vi "Fire Control.vi"(10 "ShooterDevRef":T14={"Frisbee Load Motor"={"DeviceStatus"={"status"=FALSE, "code"=0, "source"=""}, "Type"=enum."PWM", "PWM"={"Digital Module"=enum."Digital Module 1", "PWM Channel"=enum."Invalid", "DeadBand"={"Name"="", "maxPositivePwm"=0, "minPositivePwm"=0, "centerPwm"=0, "maxNegativePwm"=0, "minNegativePwm"=0, "angularRange"=0}}, "CAN"={"Device Number"=0, "Control Mode"=enum."Percent VBus", "Semaphore"=refnum, "Max Vout"=12.0}, "Invert"=FALSE, "TransformRef"=refnum, "InvTransformRef"=refnum}, "On Deck Sensor"={"DevStatus"={"status"=FALSE, "code"=0, "source"=""}, "DIO Channel"=enum."DIO 1", "Digital Module"=enum."Digital Module 1"}, "Load Sensor"={"DevStatus"={"status"=FALSE, "code"=0, "source"=""}, "DIO Channel"=enum."DIO 1", "Digital Module"=enum."Digital Module 1"}, "Front Sensor"={"DevStatus"={"status"=FALSE, "code"=0, "source"=""}, "DIO Channel"=enum."DIO 1", "Digital Module"=enum."Digital Module 1"}, "Firing Motors"={"DevStatus"={"status"=FALSE, "code"=0, "source"=""}, "Motors[]"=[], "Square Inputs"=FALSE, "Max Output"=1.0, "Isochronous"=FALSE}, "Piston"={"DevStatus"={"status"=FALSE, "code"=0, "source"=""}, "Relay Channel"=enum."Invalid", "Digital Module"=enum."Digital Module 1", "Relay Direction"=enum."Both directions"}}, 11 "Fire":bool) -> ()   [LabVIEW 2013]
uses:
  <vilib>/Rock Robotics/WPI/MotorControl/WPI_MotorControlDeviceRef.ctl
  <vilib>/Rock Robotics/SystemInterfaces/Typedef/FPGA_TypedefDigitalModule.ctl
  <vilib>/Rock Robotics/SystemInterfaces/DIO/FPGA_DIOPWMChannel.ctl
  <vilib>/Rock Robotics/WPI/PWM/WPI_PWMDeadband.ctl
  <vilib>/Rock Robotics/WPI/CAN/Jaguar/SubVIs/WPI_CANJaguar_ControlMode.ctl
  <vilib>/Rock Robotics/WPI/PWM/WPI_PWMTransform_ConPane.ctl
  <vilib>/Rock Robotics/WPI/DigitalInput/WPI_DigitalInputDevRef.ctl
  <vilib>/Rock Robotics/SystemInterfaces/DIO/FPGA_DIOChannel.ctl
  <vilib>/Rock Robotics/WPI/RobotDrive/WPI_RobotDriveDevRef.ctl
  <vilib>/Rock Robotics/WPI/Relay/WPI_RelayDevRef.ctl
  <vilib>/Rock Robotics/SystemInterfaces/DIO/FPGA_DIORelayChannel.ctl
  <vilib>/Rock Robotics/WPI/Relay/WPI_RelayDirection.ctl
  Utils/ShooterStateEnum.ctl
  <vilib>/Rock Robotics/WPI/Relay/WPI_RelayValue.ctl
panel:
  in  "Load Disk Time":dbl
  in  "Wheel Time":dbl
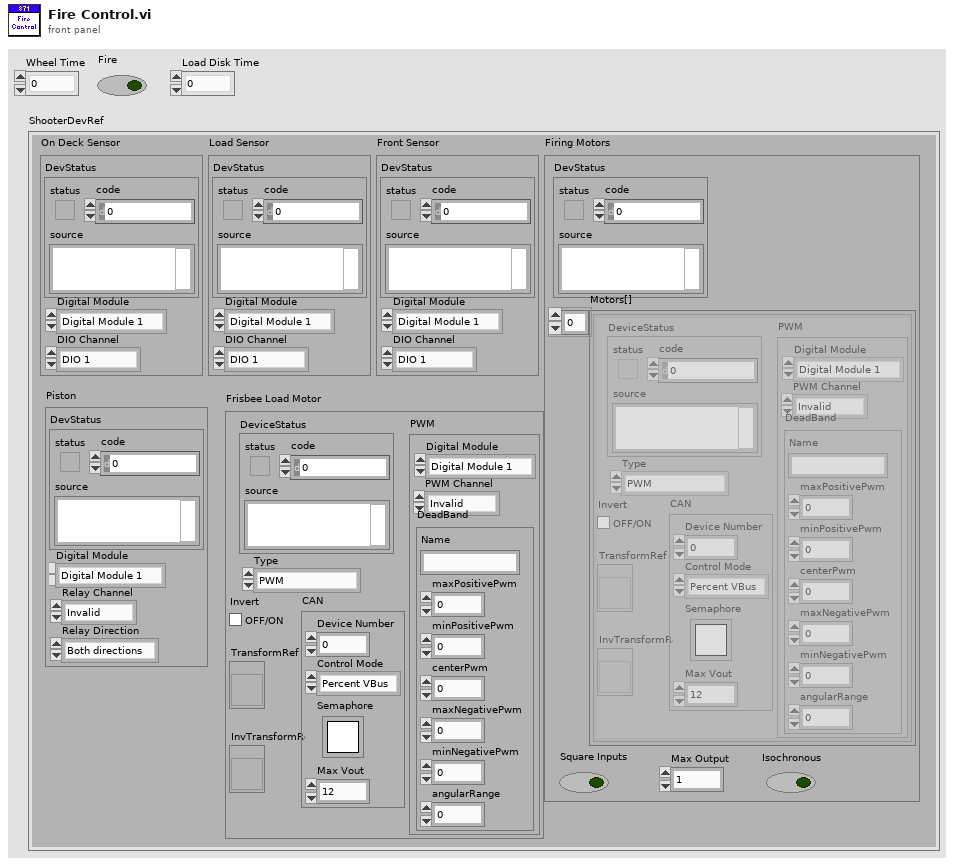
[diagram p1: front panel]
types:
  T1 = typedef "WPI_MotorControlDeviceRef.ctl" = cluster{"DeviceStatus":errorcluster, "Type":enum16{"PWM", "CAN"}, "PWM":cluster{"Digital Module":T2, "PWM Channel":T3, "DeadBand":T4}, "CAN":cluster{"Device Number":u8, "Control Mode":T5, "Semaphore":T6, "Max Vout":dbl}, "Invert":bool, "TransformRef":T7, "InvTransformRef":T7}
  T2 = typedef "FPGA_TypedefDigitalModule.ctl" = enum16{"Digital Module 1", "Digital Module 2"}
  T3 = typedef "FPGA_DIOPWMChannel.ctl" = enum8{"PWM 1", "PWM 2", "PWM 3", "PWM 4", "PWM 5", "PWM 6", "PWM 7", "PWM 8", "PWM 9", "PWM 10", "Invalid"}
  T4 = typedef "WPI_PWMDeadband.ctl" = cluster{"Name":string, "maxPositivePwm":i32, "minPositivePwm":i32, "centerPwm":i32, "maxNegativePwm":i32, "minNegativePwm":i32, "angularRange":u16}
  T5 = typedef "WPI_CANJaguar_ControlMode.ctl" = enum8{"Percent VBus", "Current", "Speed", "Position", "Voltage"}
  T6 = typedef "Semaphore RefNum" = refnum<k1>
  T7 = typedef "WPI_PWMTransform_ConPane.ctl" = refnum<vi>
  T8 = typedef "WPI_DigitalInputDevRef.ctl" = cluster{"DevStatus":errorcluster, "DIO Channel":T9, "Digital Module":T2}
  T9 = typedef "FPGA_DIOChannel.ctl" = enum8{"DIO 1", "DIO 2", "DIO 3", "DIO 4", "DIO 5", "DIO 6", "DIO 7", "DIO 8", "DIO 9", "DIO 10", "DIO 11", "DIO 12", "DIO 13", "DIO 14", "Invalid"}
  T10 = typedef "WPI_RobotDriveDevRef.ctl" = cluster{"DevStatus":errorcluster, "Motors[]":T1[], "Square Inputs":bool, "Max Output":dbl, "Isochronous":bool}
  T11 = typedef "WPI_RelayDevRef.ctl" = cluster{"DevStatus":errorcluster, "Relay Channel":T12, "Digital Module":T2, "Relay Direction":T13}
  T12 = typedef "FPGA_DIORelayChannel.ctl" = enum8{"Relay 1", "Relay 2", "Relay 3", "Relay 4", "Relay 5", "Relay 6", "Relay 7", "Relay 8", "Invalid"}
  T13 = typedef "WPI_RelayDirection.ctl" = enum16{"Both directions", "Forward only", "Reverse only"}
  T14 = cluster{"Frisbee Load Motor":T1, "On Deck Sensor":T8, "Load Sensor":T8, "Front Sensor":T8, "Firing Motors":T10, "Piston":T11}
  T15 = typedef "ShooterStateEnum.ctl" = enum16{"Load Disk", "Wait for Op", "Spin Up", "Fire Piston", "Wait For Fired", "Spin Down"}
  T16 = typedef "WPI_RelayValue.ctl" = enum16{"Off", "On", "Forward", "Reverse"}
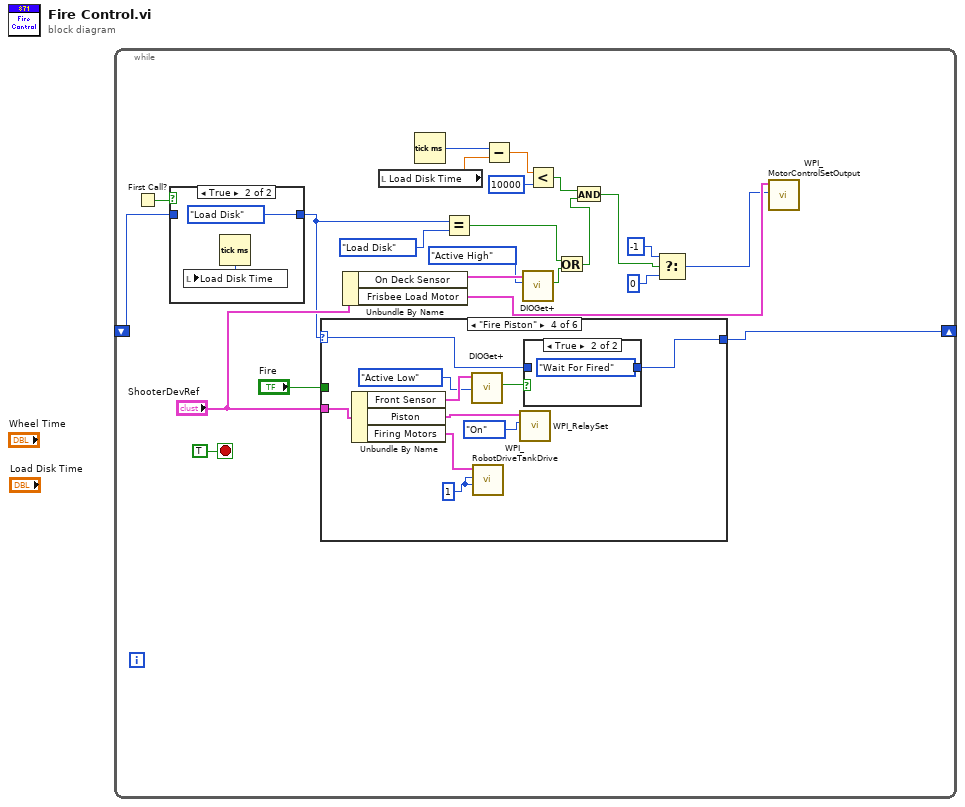
[diagram p0: block diagram]
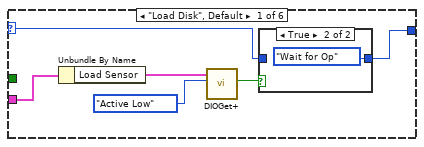
[diagram p3: hidden frame]
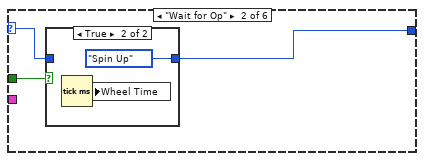
[diagram p5: hidden frame]
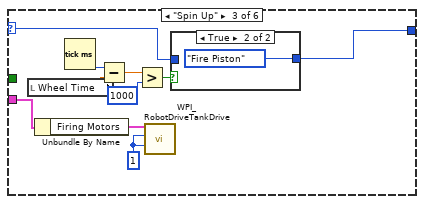
[diagram p7: hidden frame]
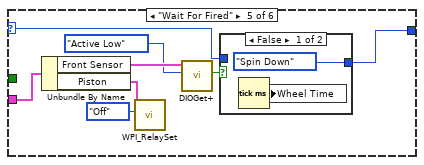
[diagram p10: hidden frame]
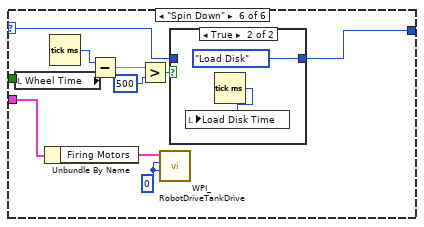
[diagram p12: hidden frame]
diagram:
  n1 = while {
    shift-right: [w19] -> _
    shift-left: _ -> [w21]
    stop <- TRUE stop-if-true
    n2 = First Call?() -> (First Call?: T/F=w22:bool)
    n3 = case shown="True" w22 {
      tunnel: [w24 ShooterStateEnum."Load Disk"] -> w13
      tunnel: w21 -> [w24 _]
      frame False {
      }
      frame True {
        n4 = Tick Count (ms)() -> (millisecond timer value=w25:u32)
        n5 = local write "Load Disk Time"(w25) -> ()
      }
    }
    n6 = case shown="\"Fire Piston\"" w13 {
      selector: w13 -> [w30 w35 w41 w60 w68 w77]
      tunnel: [w31 w36 w42 w61 w69 w78] -> w19
      tunnel: "ShooterDevRef" -> [w32 _ w50 w62 w72 w85]
      tunnel: "Fire" -> [_ w37 _ _ _ _]
      frame "Load Disk", Default {
        n7 = Unbundle By Name(w32) -> ("Load Sensor"=w29:T8)
        n8 = call "DIOGet+.vi"("Sensor Type"=enum16{"Active Low", "Active High"}."Active Low", "DigitalInputDevRefIn"=w29) -> ("Value"=w27:bool)  [unwired: 7 in, 2 out]
        n9 = case shown="True" w27 {
          tunnel: [w33 ShooterStateEnum."Wait for Op" ("Enum")] -> w31
          tunnel: w30 -> [w33 _]
          frame False {
          }
          frame True {
          }
        }
      }
      frame "Wait for Op" {
        n10 = case shown="True" w37 {
          tunnel: [w38 ShooterStateEnum."Spin Up" ("Enum")] -> w36
          tunnel: w35 -> [w38 _]
          frame False {
          }
          frame True {
            n11 = Tick Count (ms)() -> (millisecond timer value=w39:u32)
            n12 = local write "Wheel Time"(w39) -> ()
          }
        }
      }
      frame "Spin Up" {
        w48 = 1
        n13 = local read "Wheel Time"() -> (w47:dbl)
        n14 = Unbundle By Name(w50) -> ("Firing Motors"=w49:T10)
        n15 = Tick Count (ms)() -> (millisecond timer value=w46:u32)
        n16 = Subtract(x=w46, y=w47) -> (x-y=w45:dbl)
        n17 = Greater?(x=w45, y=1000) -> (0:w43:bool)
        n18 = call <vilib>:"WPI_RobotDriveTankDrive.vi"("Right axis value"=w48, "Left axis value"=w48, "RobotDriveDevRef"=w49) -> ()  [unwired: 6 in, 3 out]
        n19 = case shown="True" w43 {
          tunnel: [w51 ShooterStateEnum."Fire Piston"] -> w42
          tunnel: w41 -> [w51 _]
          frame False {
          }
          frame True {
          }
        }
      }
      frame "Fire Piston" {
        w57 = 1
        n20 = Unbundle By Name(w62) -> ("Front Sensor"=w55:T8, "Piston"=w59:T11, "Firing Motors"=w58:T10)
        n21 = call "DIOGet+.vi"("Sensor Type"=enum16{"Active Low", "Active High"}."Active Low", "DigitalInputDevRefIn"=w55) -> ("Value"=w54:bool)  [unwired: 7 in, 2 out]
        n22 = call <vilib>:"WPI_RobotDriveTankDrive.vi"("Right axis value"=w57, "Left axis value"=w57, "RobotDriveDevRef"=w58) -> ()  [unwired: 6 in, 3 out]
        n23 = call <vilib>:"WPI_RelaySet.vi"("RelayValue"=WPI_RelayValue."On", "RelayDevRef"=w59) -> ()  [unwired: 8 in, 2 out]
        n24 = case shown="True" w54 {
          tunnel: [w63 ShooterStateEnum."Wait For Fired"] -> w61
          tunnel: w60 -> [w63 _]
          frame False {
          }
          frame True {
          }
        }
      }
      frame "Wait For Fired" {
        n25 = Unbundle By Name(w72) -> ("Front Sensor"=w67:T8, "Piston"=w70:T11)
        n26 = call <vilib>:"WPI_RelaySet.vi"("RelayValue"=WPI_RelayValue."Off", "RelayDevRef"=w70) -> ()  [unwired: 8 in, 2 out]
        n27 = call "DIOGet+.vi"("Sensor Type"=enum16{"Active Low", "Active High"}."Active Low", "DigitalInputDevRefIn"=w67) -> ("Value"=w66:bool)  [unwired: 7 in, 2 out]
        n28 = case shown="False" w66 {
          tunnel: [ShooterStateEnum."Spin Down" w75] -> w69
          tunnel: w68 -> [_ w75]
          frame False {
            n29 = Tick Count (ms)() -> (millisecond timer value=w73:u32)
            n30 = local write "Wheel Time"(w73) -> ()
          }
          frame True {
          }
        }
      }
      frame "Spin Down" {
        w83 = 0
        n31 = local read "Wheel Time"() -> (w76:dbl)
        n32 = Unbundle By Name(w85) -> ("Firing Motors"=w84:T10)
        n33 = Tick Count (ms)() -> (millisecond timer value=w82:u32)
        n34 = Subtract(x=w82, y=w76) -> (x-y=w81:dbl)
        n35 = Greater?(x=w81, y=500) -> (0:w79:bool)
        n36 = call <vilib>:"WPI_RobotDriveTankDrive.vi"("Right axis value"=w83, "Left axis value"=w83, "RobotDriveDevRef"=w84) -> ()  [unwired: 6 in, 3 out]
        n37 = case shown="True" w79 {
          tunnel: [w86 ShooterStateEnum."Load Disk"] -> w78
          tunnel: w77 -> [w86 _]
          frame False {
          }
          frame True {
            n38 = Tick Count (ms)() -> (millisecond timer value=w87:u32)
            n39 = local write "Load Disk Time"(w87) -> ()
          }
        }
      }
    }
    n40 = Unbundle By Name("ShooterDevRef") -> ("On Deck Sensor"=w3:T8, "Frisbee Load Motor"=w9:T1)
    n41 = local read "Load Disk Time"() -> (w17:dbl)
    n42 = Tick Count (ms)() -> (millisecond timer value=w18:u32)
    n43 = Equal?(x=w13, y=ShooterStateEnum."Load Disk") -> (x = y?=w7:bool)
    n44 = Subtract(x=w18, y=w17) -> (x-y=w16:dbl)
    n45 = call "DIOGet+.vi"("Sensor Type"=enum16{"Active Low", "Active High"}."Active High", "DigitalInputDevRefIn"=w3) -> ("Value"=w2:bool)  [unwired: 7 in, 2 out]
    n46 = Less?(x=w16, y=10000) -> (x < y?=w5:bool)
    n47 = Or(x=w7, y=w2) -> (x .or. y?=w6:bool)
    n48 = And(x=w5, y=w6) -> (x .and. y?=w4:bool)
    n49 = Select(t=-1, s=w4, f=0) -> (s? t:f=w8:i32)
    n50 = call <vilib>:"WPI_MotorControlSetOutput.vi"("Output"=w8, "MotorControlDevRef"=w9) -> ()  [unwired: 7 in, 3 out]
  }
